vi "TPG261_MeasData.vi"(8 "Fehler (Eingang)":errorcluster, 11 "Referenz in":refnum<visa-resource-name>) -> (0 "Cluster (Ausgang)":errorcluster, 2 "Pressure CH1":dbl format="%.3e", 3 "Referenz out":refnum<visa-resource-name>, 5 "Status CH1":i32(ring) items=["data OK", "underrange", "overrange", "sensor error", "sensor off", "no sensor", "ID error"])   [LabVIEW 2012]
doc: "PRX - Measurement Data Gauges 1 and 2\n\nReceive: a,sx.xxxxEsxx,b,sy.yyyyEsyy\n\nStatus gauge 1,\na =\n0 –> Measurement data okay\n1 –> Underrange\n2 –> Overrange\n3 –> Sensor error\n4 –> Sensor off (IKR, PKR, IMR, PBR)\n5 –> No sensor (output: 5,2.0000E-2 [hPa])\n6 –> Identification error\nMeasurement value gauge 1 [in current pressure unit]\nStatus gauge 2,\nb= \nMeasurement value gauge 2 [in current pressure unit]\n\nValues always in exponential format.\nFor logarithmic gauges, the 3rd and 4th decimal are always 0."
uses:
  <instrlib>/PV ActiveLine/PV ActiveLine.lvlib
panel:
  out "String Out":string
  out "Array Out":string[](array[string])
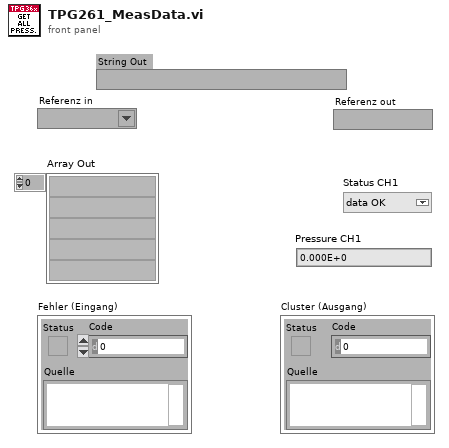
[diagram p1: front panel]
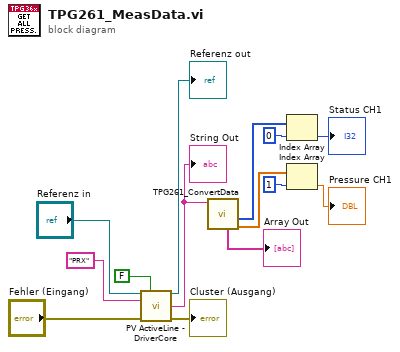
[diagram p0: block diagram]
diagram:
  n1 = call <instrlib>:"PV ActiveLine - DriverCore.vi"("Referenz in"="Referenz in", "Write/Read"=FALSE, "Command"="PRX", "Fehler (Eingang)"="Fehler (Eingang)") -> ("Referenz out"=→"Referenz out":refnum<visa-resource-name>, "String Out"=w8:string, "Cluster (Ausgang)"=→"Cluster (Ausgang)":errorcluster)  [unwired: 9 in]
  "String Out" <- w8
  n2 = call "TPG261_ConvertData.vi"("String in"=w8) -> ("DBL out"=w1:dbl[], "Integer Out"=w2:i32[], "Array"=→"Array Out":string[])  [unwired: 6 in, 2 out]
  n3 = Index Array(array=w2, index=0 ("Index")) -> (element=→"Status CH1":i32)
  n4 = Index Array(array=w1, index=1 ("Index")) -> (element=→"Pressure CH1":dbl)
